vi "DAQgenV4.vi"() -> ()   [LabVIEW 2017]
uses:
  <vilib>/rvi/Emulation/niFpgaGetClockAttributes.vi
  <vilib>/rvi/Emulation/niFpgaSctlEmulationGetInTimedLoop.vi
  <vilib>/rvi/Emulation/niFpgaEmulationReportErrorSimple.vi
  <vilib>/rvi/eio/common/nirviEmuTemplateMethod_errors.vi
  <vilib>/rvi/interface/RandomDataEmulation/niFpgaRandomDataHandleErrors.vi
  <vilib>/rvi/Emulation/niFpgaCriticalErrorInLSC.vi
  <vilib>/eio/EIONode/EIONode.xnode
  <vilib>/rvi/DataTransferAndStorage/Container/XNode/niFpgaContainer.xnode
  <vilib>/rvi/interface/RandomDataEmulation/nirviRandomDataFpgaReadWriteTemplate.vi
panel:
  in  "Wavegen!":bool
  in  "Count(Ticks)":u32=500000
  in  "stop":bool
  in  "Sampling Rate (Hz)":i16=1000
  in  "# Samples":i16=10000
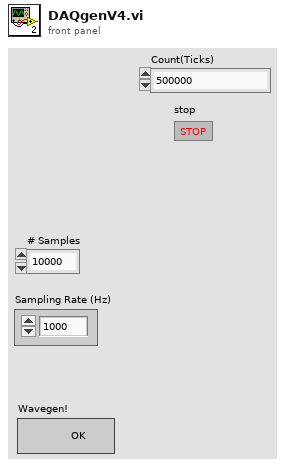
[diagram p1: front panel]
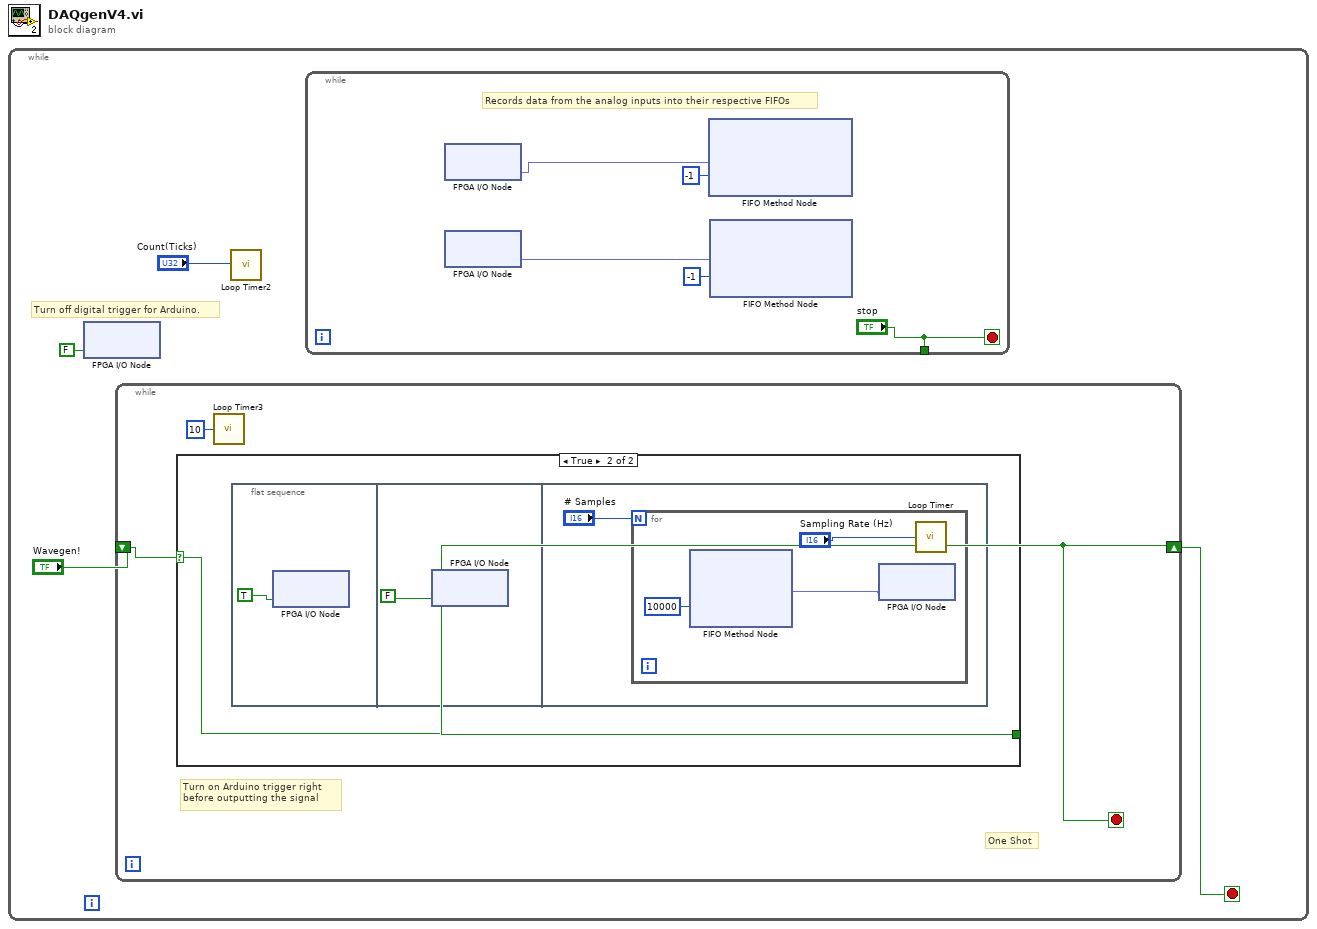
[diagram p0: block diagram]
diagram:
  n1 = while {
    stop <- w2 stop-if-true
    # "Turn off digital trigger for Arduino."
    n2 = xnode "FPGA I/O Node"("DIO0"=FALSE) -> ()  [unwired: 1 in, 1 out]
    n3 = while {
      shift-right: [w10] -> w2
      shift-left: "Wavegen!" -> [w12]
      stop <- w10 stop-if-true
      # "Turn on Arduino trigger right \nbefore outputting the signal"
      # "One Shot"
      n4 = case shown="True" w12 {
        selector: w12 -> [w13 w14]
        tunnel: [w13 w14] -> w10
        frame False {
        }
        frame True {
          n5 = flat-sequence {
            frame #0 {
              n6 = xnode "FPGA I/O Node"("DIO0"=TRUE) -> ()  [unwired: 1 in, 1 out]
            }
            frame #1 {
              n7 = xnode "FPGA I/O Node"("DIO0"=FALSE) -> ()  [unwired: 1 in, 1 out]
            }
            frame #2 {
              n8 = for {
                N: "# Samples" -> [_]
                n9 = xnode ("FIFO Method Node")("Timeout"=10000) -> ("Element"=w18:fxp<+,16,3>)  [unwired: 1 in, 2 out]
                n10 = xnode "FPGA I/O Node"("AO0"=w18) -> ()  [unwired: 1 in, 1 out]
                n11 = call "Loop Timer"("Count(Ticks)"="Sampling Rate (Hz)") -> ()  [unwired: 1 out]
              }
            }
          }
        }
      }
      n12 = call "Loop Timer3"("Count(Ticks)"=u32 10) -> ()  [unwired: 1 out]
    }
    n13 = call "Loop Timer2"("Count(Ticks)"="Count(Ticks)") -> ()  [unwired: 1 out]
    n14 = while {
      tunnel: ["stop"] -> _
      stop <- "stop" stop-if-true
      # "Records data from the analog inputs into their respective FIFOs"
      n15 = xnode "FPGA I/O Node"() -> ("AI0"=w6:fxp<+,16,3>)  [unwired: 1 in, 1 out]
      n16 = xnode "FPGA I/O Node"() -> ("AI7"=w5:fxp<+,16,3>)  [unwired: 1 in, 1 out]
      n17 = xnode ("FIFO Method Node")("Element"=w6, "Timeout"=-1) -> ()  [unwired: 1 in, 2 out]
      n18 = xnode ("FIFO Method Node")("Element"=w5, "Timeout"=-1) -> ()  [unwired: 1 in, 2 out]
    }
  }
